vi "Main.vi"() -> ()   [LabVIEW 2011]
panel:
  in  "09":bool
  in  "08":bool
  in  "07":bool
  in  "06":bool
  in  "05":bool
  in  "04":bool
  in  "03":bool
  in  "02":bool
  out "number (0 to 1)":dbl
  in  "stop":bool
  in  "01":bool
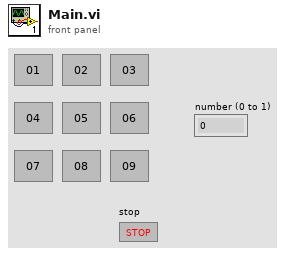
[diagram p1: front panel]
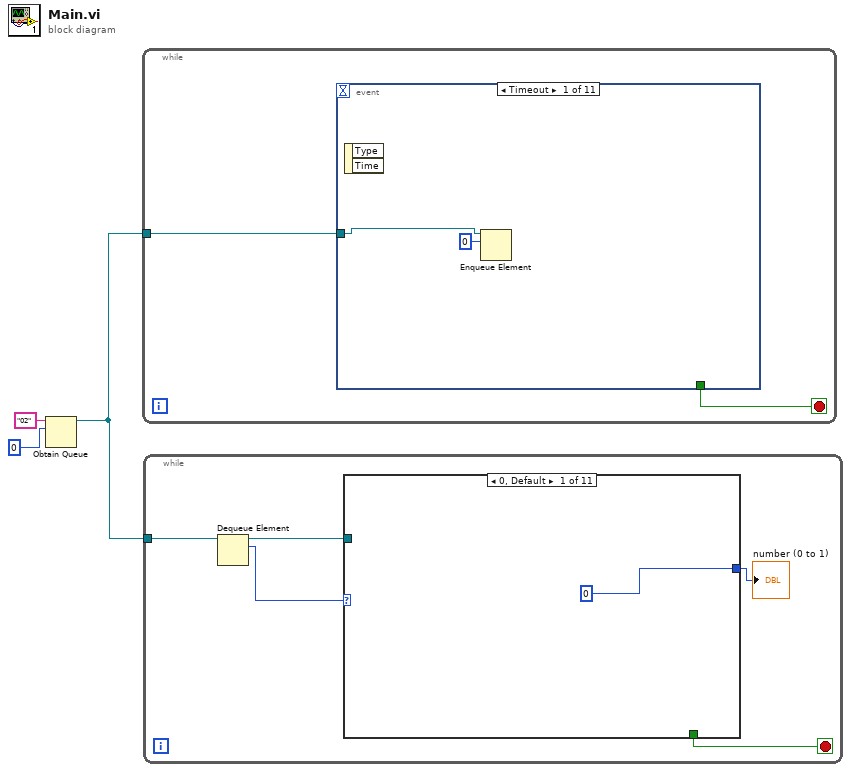
[diagram p0: block diagram]
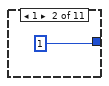
[diagram p2: hidden frame]
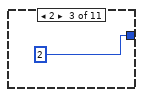
[diagram p3: hidden frame]
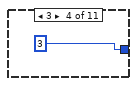
[diagram p4: hidden frame]
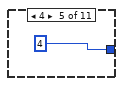
[diagram p5: hidden frame]
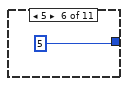
[diagram p6: hidden frame]
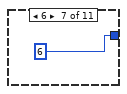
[diagram p7: hidden frame]
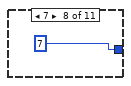
[diagram p8: hidden frame]
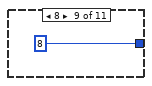
[diagram p9: hidden frame]
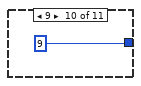
[diagram p10: hidden frame]
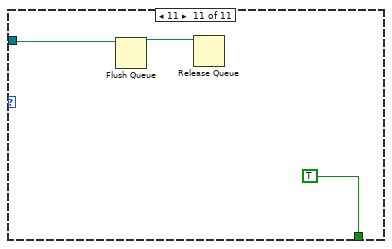
[diagram p11: hidden frame]
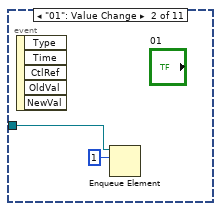
[diagram p12: hidden frame]
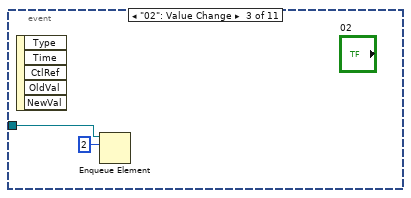
[diagram p13: hidden frame]
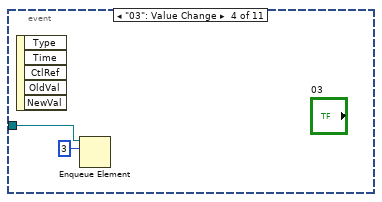
[diagram p14: hidden frame]
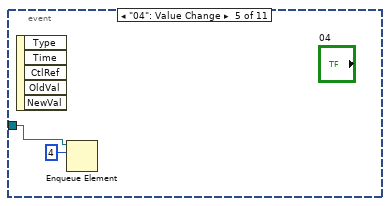
[diagram p15: hidden frame]
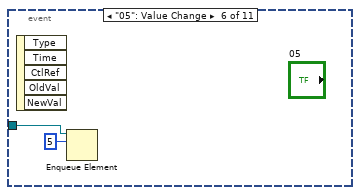
[diagram p16: hidden frame]
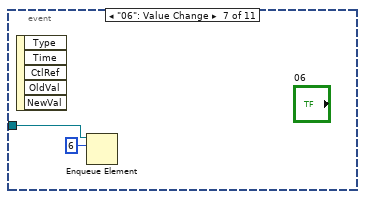
[diagram p17: hidden frame]
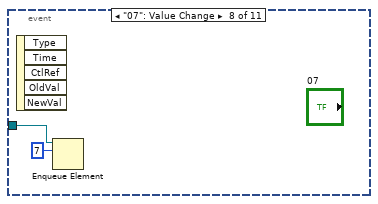
[diagram p18: hidden frame]
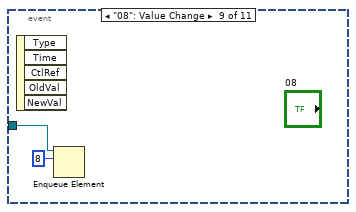
[diagram p19: hidden frame]
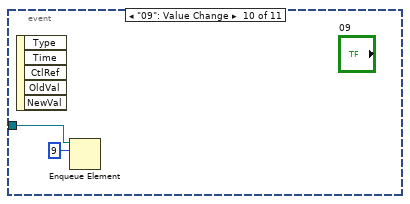
[diagram p20: hidden frame]
diagram:
  n1 = Obtain Queue(name (unnamed)="02", element data type=0) -> (queue out=w2:refnum<queue>)  [unwired: 3 in, 2 out]
  n2 = while {
    tunnel: w2 -> [w5]
    stop <- w4 stop-if-true
    n3 = event shown="[0] Timeout" {
      selector: _ -> [_ _ _ _ _ _ _ _ _ _ _]
      dyn-events: _ -> [_ _ _ _ _ _ _ _ _ _ _]
      timeout: _ -> [_ _ _ _ _ _ _ _ _ _ _]
      tunnel: w5 -> [w6 w9 w10 w12 w14 w16 w18 w20 w22 w24 w28]
      tunnel: [_ _ _ _ _ _ _ _ _ _ TRUE] -> w4
      event Timeout {
        n4 = event-data() -> ()  [unwired: 1 in, 2 out]
        n5 = Enqueue Element(queue=w6, element=0) -> ()  [unwired: 2 in, 3 out]
      }
      event "01": Value Change {
        n6 = event-data() -> ()  [unwired: 1 in, 5 out]
        n7 = Enqueue Element(queue=w9, element=1) -> ()  [unwired: 2 in, 3 out]
      }
      event "02": Value Change {
        n8 = event-data() -> ()  [unwired: 1 in, 5 out]
        n9 = Enqueue Element(queue=w10, element=2) -> ()  [unwired: 2 in, 3 out]
      }
      event "03": Value Change {
        n10 = event-data() -> ()  [unwired: 1 in, 5 out]
        n11 = Enqueue Element(queue=w12, element=3) -> ()  [unwired: 2 in, 3 out]
      }
      event "04": Value Change {
        n12 = event-data() -> ()  [unwired: 1 in, 5 out]
        n13 = Enqueue Element(queue=w14, element=4) -> ()  [unwired: 2 in, 3 out]
      }
      event "05": Value Change {
        n14 = event-data() -> ()  [unwired: 1 in, 5 out]
        n15 = Enqueue Element(queue=w16, element=5) -> ()  [unwired: 2 in, 3 out]
      }
      event "06": Value Change {
        n16 = event-data() -> ()  [unwired: 1 in, 5 out]
        n17 = Enqueue Element(queue=w18, element=6) -> ()  [unwired: 2 in, 3 out]
      }
      event "07": Value Change {
        n18 = event-data() -> ()  [unwired: 1 in, 5 out]
        n19 = Enqueue Element(queue=w20, element=7) -> ()  [unwired: 2 in, 3 out]
      }
      event "08": Value Change {
        n20 = event-data() -> ()  [unwired: 1 in, 5 out]
        n21 = Enqueue Element(queue=w22, element=8) -> ()  [unwired: 2 in, 3 out]
      }
      event "09": Value Change {
        n22 = event-data() -> ()  [unwired: 1 in, 5 out]
        n23 = Enqueue Element(queue=w24, element=9) -> ()  [unwired: 2 in, 3 out]
      }
      event "stop": Value Change {
        n24 = event-data() -> ()  [unwired: 1 in, 5 out]
        n25 = Enqueue Element(queue=w28, element=11) -> ()  [unwired: 2 in, 3 out]
      }
    }
  }
  n26 = while {
    tunnel: w2 -> [w33]
    stop <- w31 stop-if-true
    n27 = Dequeue Element(queue=w33) -> (queue out=w30:refnum<queue>, element=w32:i32)  [unwired: 2 in, 2 out]
    n28 = case shown="0, Default" w32 {
      tunnel: [_ _ _ _ _ _ _ _ _ _ TRUE] -> w31
      tunnel: w30 -> [_ _ _ _ _ _ _ _ _ _ w45]
      tunnel: [0 ("element") 1 ("element") 2 ("element") 3 ("element") 4 ("element") 5 ("element") 6 ("element") 7 ("element") 8 ("element") 9 ("element") _] -> w29
      frame 0, Default {
      }
      frame 1 {
      }
      frame 2 {
      }
      frame 3 {
      }
      frame 4 {
      }
      frame 5 {
      }
      frame 6 {
      }
      frame 7 {
      }
      frame 8 {
      }
      frame 9 {
      }
      frame 11 {
        n29 = Flush Queue(queue=w45) -> (queue out=w46:refnum<queue>)  [unwired: 1 in, 2 out]
        n30 = Release Queue(queue=w46) -> ()  [unwired: 2 in, 3 out]
      }
    }
    "number (0 to 1)" <- w29
  }
